vi "Case Structures.vi"() -> ()   [LabVIEW 2018]
panel:
  out "A+B":dbl
  out "A/B":dbl
  out "A*B":dbl
  in  "Case":dbl
  out "A-B":dbl
  in  "B":dbl
  in  "A":dbl
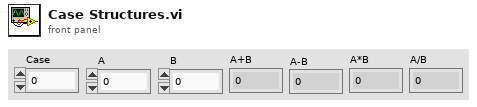
[diagram p1: front panel]
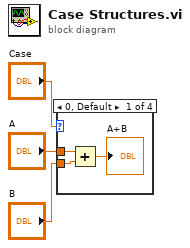
[diagram p0: block diagram]
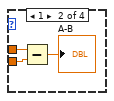
[diagram p2: hidden frame]
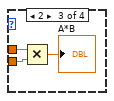
[diagram p3: hidden frame]
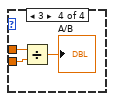
[diagram p4: hidden frame]
diagram:
  n1 = case shown="0, Default" "Case" {
    tunnel: "A" -> [w6 w9 w12 w15]
    tunnel: "B" -> [w5 w8 w11 w14]
    frame 0, Default {
      n2 = Add(x=w6, y=w5) -> (x+y=→"A+B":dbl)
    }
    frame 1 {
      n3 = Subtract(x=w9, y=w8) -> (x-y=→"A-B":dbl)
    }
    frame 2 {
      n4 = Multiply(x=w12, y=w11) -> (x*y=→"A*B":dbl)
    }
    frame 3 {
      n5 = Divide(x=w15, y=w14) -> (x/y=→"A/B":dbl)
    }
  }
